vi "randomize.vi"(6 "Test":T1, 11 "Test Data in":T2) -> (2 "encoded packets":string[](array[string]), 3 "Test Data out":T2)   [LabVIEW 2024, in "EncodingTester.lvlib"]
uses:
  EncodingTester.lvlib
  Tests/test_data--cluster.ctl
  Tests/packetized_data--cluster.ctl
  Tests/tests--enum.ctl
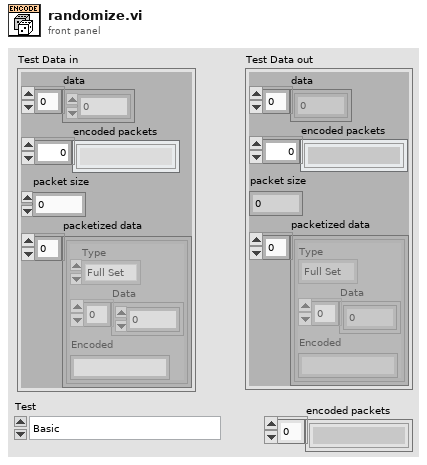
[diagram p1: front panel]
types:
  T1 = typedef "EncodingTester.lvlib/tests--enum.ctl" = enum16{"Basic", "Pre-Allocated", "Packet-Type Case", "No IPE"}
  T2 = typedef "EncodingTester.lvlib/test_data--cluster.ctl" = cluster{"data":dbl[], "encoded packets":string[], "packet size":i32, "packetized data":T3[]}
  T3 = typedef "EncodingTester.lvlib/packetized_data--cluster.ctl" = cluster{"Type":enum16{"Full Set", "Last Set"}, "Data":dbl[], "Encoded":string}
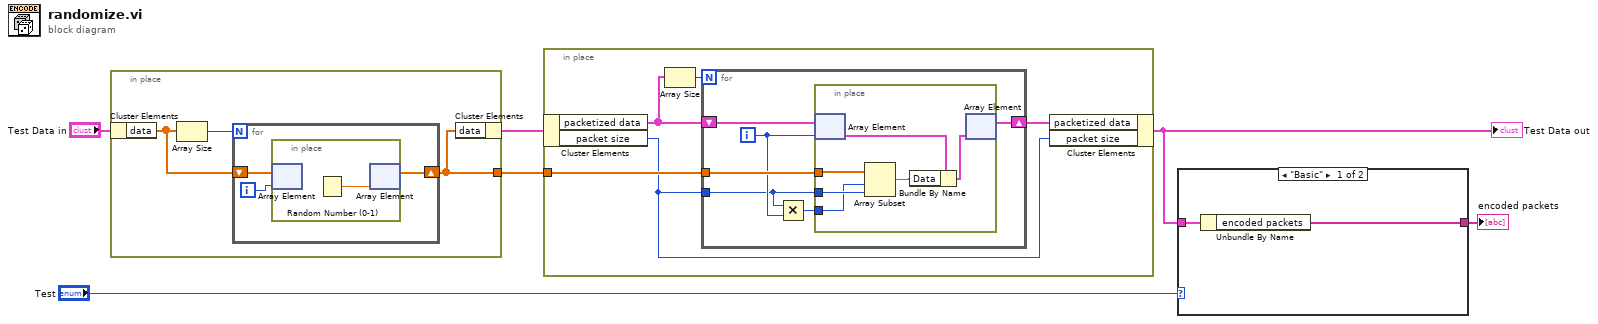
[diagram p0: block diagram]
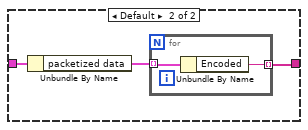
[diagram p2: hidden frame]
diagram:
  n1 = in-place {
    in-place-border: [w7] -> w4
    n2 = in-place-cluster #1("Test Data in") -> ("data"=w8:dbl[])
    n3 = Array Size(array=w8) -> (size(s)=w9:i32)
    n4 = for {
      N: w9 -> [_]
      shift-right: [w10] -> w7
      shift-left: w8 -> [w12]
      i -> [w11]
      n5 = in-place {
        n6 = in-place-array #2(w12, w11) -> ()  [unwired: 1 out]
        n7 = Random Number (0-1)() -> (number: 0 to 1=w13:dbl)
        n8 = in-place-array #2(w13) -> (w10:dbl[])  [unwired: 1 out]
      }
    }
    n9 = in-place-cluster #1("data"=w7) -> (w5:T2)
  }
  n10 = in-place {
    in-place-border: w4 -> [w15]
    n11 = in-place-cluster #3(w5) -> ("packetized data"=w17:T3[], "packet size"=w14:i32)
    n12 = Array Size(array=w17) -> (size(s)=w18:i32)
    n13 = for {
      N: w18 -> [_]
      shift-right: [w23] -> w16
      shift-left: w17 -> [w24]
      tunnel: w15 -> [w22]
      tunnel: w14 -> [w20]
      i -> [w21]
      n14 = Multiply(x=w20, y=w21) -> (x*y=w19:i32)
      n15 = in-place {
        in-place-border: w22 -> [w30]
        in-place-border: w20 -> [w29]
        in-place-border: w19 -> [w28]
        n16 = in-place-array #4(w24, w21) -> (w27:T3)
        n17 = Array Subset(array=w30, index=w28, length=w29) -> (w26:dbl[])
        n18 = Bundle By Name(cluster=w27, "Data"=w26) -> (w25:T3)
        n19 = in-place-array #4(w25) -> (w23:T3[])  [unwired: 1 out]
      }
    }
    n20 = in-place-cluster #3("packetized data"=w16, "packet size"=w14) -> (w2:T2)
  }
  "Test Data out" <- w2
  n21 = case shown="\"Basic\"" "Test" {
    tunnel: w2 -> [w32 w35]
    tunnel: [w31 w33] -> w1
    frame "Basic" {
      n22 = Unbundle By Name(w32) -> ("encoded packets"=w31:string[])
    }
    frame Default {
      n23 = Unbundle By Name(w35) -> ("packetized data"=w34:T3[])
      n24 = for {
        tunnel: w34 -> [w37] mode=indexing
        tunnel: [w36] -> w33 mode=indexing
        n25 = Unbundle By Name(w37) -> ("Encoded"=w36:string)
      }
    }
  }
  "encoded packets" <- w1
